vi "SimplePackUnpack.vi"() -> ()   [LabVIEW 2019]
uses:
  labview source/gRPC lv Support/Server API/typeDefs/Message Metadata.ctl
  labview source/gRPC lv Support/Server API/typeDefs/Message Element Metadata.ctl
  labview source/gRPC lv Support/Server API/typeDefs/Message Element Type.ctl
  7fd04eb5-0132-428e-93dc-a7bf2da436d2.vi
  487e9c1f-f261-4604-8385-308564aa59d5.vi
  labview source/gRPC lv Support/Server API/Translate Protobuf Error.vi
  <vilib>/AdvancedString/1D String Array to Delimited String.vi
  labview source/gRPC lv Support/Server API/Server/Get Server DLL Path.vi
  labview source/gRPC lv Support/grpc-lvsupport.lvlib
panel:
  out "error out":errorcluster
  out "Numeric":i32
  out "x = y?":bool
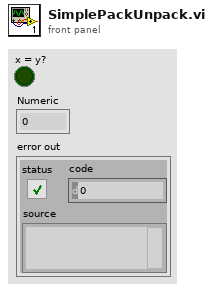
[diagram p1: front panel]
types:
  T1 = typedef "grpc-lvsupport.lvlib/Message Metadata.ctl" = cluster{"Version":i32, "Name":string, "Type Url":string, "Elements":T2[]}
  T2 = typedef "grpc-lvsupport.lvlib/Message Element Metadata.ctl" = cluster{"Embedded Message Name":string, "Protobuf Index":i32, "MessageElementType":T3, "Repeated":bool}
  T3 = typedef "grpc-lvsupport.lvlib/Message Element Type.ctl" = enum32{"Int32Value", "FloatValue", "DoubleValue", "BoolValue", "StringValue", "MessageValue", "Int64Value", "UInt32Value", "UInt64Value", "EnumValue", "Bytes", "Fixed64", "Fixed32", "SFixed64", "SFixed32", "SInt64", "SInt32"}
  T4 = typedef "grpc-lvsupport.lvlib/grpcId.ctl" = u64
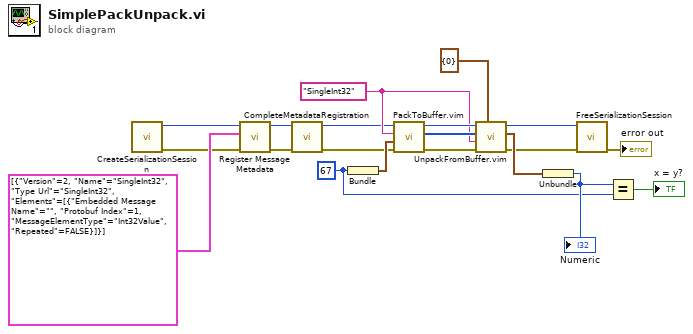
[diagram p0: block diagram]
diagram:
  w10 = 67
  w13 = "SingleInt32" ("Message Type")
  n1 = call "CreateSerializationSession.vi"() -> ("error out"=w6:errorcluster, "Serialization Session ID"=w20:T4)  [unwired: 10 in]
  n2 = call "Register Message Metadata.vi"("error in"=w6, "Messages"=T1[] [{"Version"=2, "Name"="SingleInt32", "Type Url"="SingleInt32", "Elements"=[{"Embedded Message Name"="", "Protobuf Index"=1, "MessageElementType"=enum."Int32Value", "Repeated"=FALSE}]}], "gRPCid in"=w20) -> ("error out"=w5:errorcluster, "gRPCid out"=w8:T4)  [unwired: 7 in]
  n3 = call "CompleteMetadataRegistration.vi"("error in"=w5, "gRPC ID in"=w8) -> ("error out"=w4:errorcluster, "gRPC ID Out"=w7:T4)  [unwired: 8 in]
  n4 = Bundle(w10) -> (w18:cluster{i32})  [unwired: 1 in]
  n5 = call "PackToBuffer.vim"("error in"=w4, "Data To Pack"=w18, "Message Type"=w13, "gRPCid in"=w7) -> ("error out"=w3:errorcluster, "Buffer"=w14:u8[], "gRPCid out"=w17:u64)  [unwired: 5 in]
  n6 = call "UnpackFromBuffer.vim"("Data Type"=cluster{i32} {0}, "error in"=w3, "Message Type"=w13, "Buffer"=w14, "gRPCid in"=w17) -> ("error out"=w2:errorcluster, "Unpacked Value"=w12:cluster{i32}, "gRPCid out"=w16:u64)  [unwired: 4 in]
  n7 = Unbundle(w12) -> (w11:i32)
  "Numeric" <- w11
  n8 = call "FreeSerializationSession.vi"("error in"=w2, "Serialization Session ID"=w16) -> ("error out"=→"error out":errorcluster)  [unwired: 9 in]
  n9 = Equal?(x=w11, y=w10) -> (x = y?=→"x = y?":bool)
